vi "CreateDesiredString.vi"(11 "desired":cluster{"X":dbl, "Y":dbl, "Z":dbl}) -> (3 "cmds":string[][](array[string]))   [LabVIEW 2023]
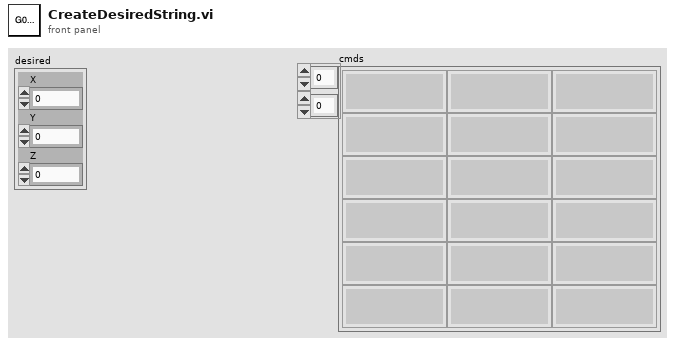
[diagram p1: front panel]
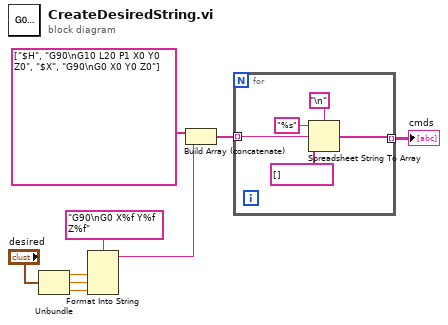
[diagram p0: block diagram]
diagram:
  n1 = Unbundle("desired") -> ("X"=w4:dbl, "Y"=w7:dbl, "Z"=w6:dbl)
  n2 = Format Into String(format string="G90\nG0 X%f Y%f Z%f" ("Value (Signaling)"), w4, w7, w6) -> (resulting string=w9:string)  [unwired: 2 in, 1 out]
  n3 = Build Array (concatenate)(string[] ["$H", "G90\nG10 L20 P1 X0 Y0 Z0", "$X", "G90\nG0 X0 Y0 Z0"], w9) -> (w2:string[])
  n4 = for {
    tunnel: w2 -> [w11] mode=indexing
    tunnel: [w10] -> w1 mode=indexing
    n5 = Spreadsheet String To Array(delimiter (Tab)="\n", format string="%s", spreadsheet string=w11, array type (2D Dbl)=string[] []) -> (array=w10:string[])
  }
  "cmds" <- w1
